vi "WriteToLog.vi"(8 "Error In":errorcluster, 9 "Data":string, 10 "Source":string, 11 "Queue In":refnum<queue>) -> (0 "Error Out":errorcluster, 3 "Queue Out":refnum<queue>)   [LabVIEW 2016]
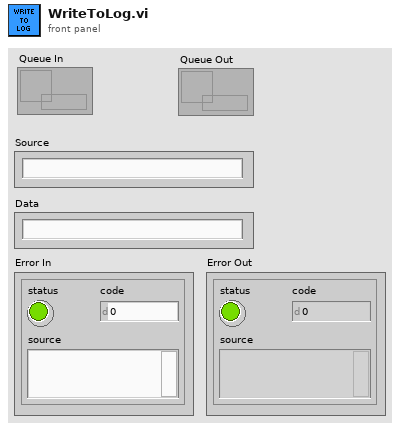
[diagram p1: front panel]
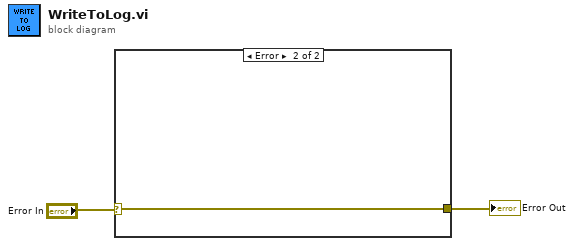
[diagram p0: block diagram]
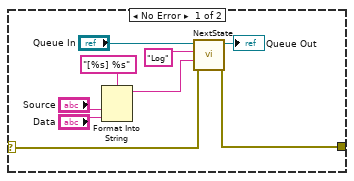
[diagram p2: hidden frame]
diagram:
  n1 = case shown="Error" "Error In" {
    selector: "Error In" -> [w4 w12]
    tunnel: [w3 w12] -> w1
    frame No Error {
      n2 = Format Into String(format string="[%s] %s" ("string"), "Source", "Data") -> (resulting string=w5:string)  [unwired: 2 in, 1 out]
      n3 = call "NextState.vi"("Error In"=w4, "Data"=w5, "State"="Log", "Queue In"="Queue In") -> ("Error Out"=w3:errorcluster, "Queue Out"=→"Queue Out":refnum<queue>)  [unwired: 6 in]
    }
    frame Error {
    }
  }
  "Error Out" <- w1
